vi "Actor.vi"(4 "Async Elements":refnum<class "Async Elements.lvclass">, 7 "Actor in":refnum<class "Actor.lvclass">) -> (0 "Error out":errorcluster, 5 "Actor out":refnum<class "Actor.lvclass">)   [LabVIEW 2020, in "jettl.lvlib"]
uses:
  jettl.lvlib
  Actor/Actor.lvclass
  Async Elements/Async Elements.lvclass
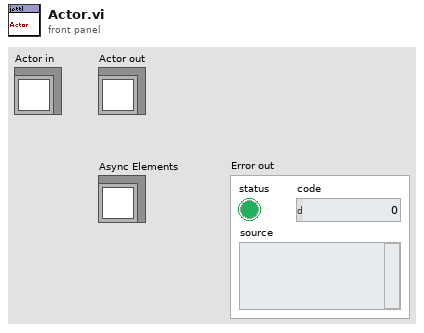
[diagram p1: front panel]
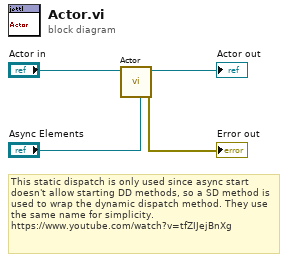
[diagram p0: block diagram]
diagram:
  # "This static dispatch is only used since async start doesn't allow starting DD methods, so a SD method is used to wrap the dynamic dispatch method. They use the same name for simplicity.\nhttps://www.youtube.com/watch?v=tfZIJejBnXg"
  n1 = call-dynamic "Actor.vi"("Async Elements"="Async Elements", "Actor in"="Actor in") -> ("Error out"=→"Error out":errorcluster, "Actor out"=→"Actor out":refnum<class "Actor.lvclass">)  [unwired: 8 in]
